vi "Inspect Modules.vi"(7 "Console Log in":refnum<class "Console Log.lvclass">, 8 "error in":errorcluster, 11 "Potting Procedure in":refnum<class "Potting Procedure.lvclass">) -> (0 "error out":errorcluster, 3 "Potting Procedure out":refnum<class "Potting Procedure.lvclass">, 5 "Console Log out":refnum<class "Console Log.lvclass">)   [LabVIEW 2011, in "Potting Procedure.lvclass"]
uses:
  Potting Procedure.lvclass
  Application Utilities/Console Log/Console Log.lvclass
  Type Definitions/Inspect Modules.ctl
  Type Definitions/Inspect Modules - Module.ctl
  Shared Components/Utils/Type Definitions/Multi-Fiducial Image.ctl
  Shared Components/Utils/Type Definitions/Physical Image.ctl
  Shared Components/Vec3d Class/Vec3d Class.lvclass
  <vilib>/vision/Image Controls.llb/IMAQ Image.ctl
  Shared Components/Utils/Type Definitions/Fiducial with Source.ctl
  Shared Components/Utils/Type Definitions/Fiducial Image.ctl
  Shared Components/Gantry Class/Gantry Class.lvclass
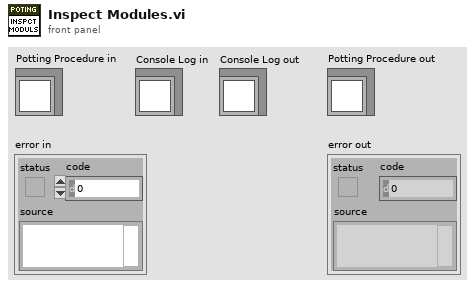
[diagram p1: front panel]
types:
  T1 = typedef "Inspect Modules.ctl" = cluster{"Has Been Run?":bool, "Module Positions":T2[]}
  T2 = typedef "Inspect Modules - Module.ctl" = cluster{"TBM-TBM":T3, "TBM-HDI":T3, "Address Pads":T3, "HDI Bond Pad References":T7[], "BBM Bond Pad References":T7[], "HV-HDI":T7, "HV-BBM":T7, "Chuck":i32, "Slot":i32, "Potting Selection":cluster{"HDI Bond Pads":bool[], "BBM Bond Pads":bool[], "TBM Inner":cluster{"Top":bool, "Left":bool, "Bottom":bool, "Right":bool}, "TBM Outer":cluster{"Top":bool, "Left":bool, "Bottom":bool, "Right":bool}, "Address Pads":cluster{"Top":bool, "Bottom":bool}, "High Voltage":cluster{"HDI":bool, "BBM":bool}}}
  T3 = typedef "Multi-Fiducial Image.ctl" = cluster{"Fiducial Image":T4, "Fiducials":cluster{"Selected Fiducial":T6, "fiducial name":string}[]}
  T4 = typedef "Physical Image.ctl" = cluster{"Image Position":refnum<class "Vec3d Class.lvclass">, "Image Reference":T5, "Field of View":cluster{"x(mm)":dbl, "y(mm)":dbl}}
  T5 = typedef "IMAQ Image.ctl" = refnum<image>
  T6 = typedef "Fiducial with Source.ctl" = cluster{"Fiducial Image Coordinate":refnum<class "Vec3d Class.lvclass">, "Fiducial Source":enum16{"Pattern Recognition", "User", "Error", "Default"}}
  T7 = typedef "Fiducial Image.ctl" = cluster{"Fiducial Image":T4, "Selected Fiducial":T6, "fiducial name":string}
  T8 = typedef "Inspect Fiducials.ctl" = cluster{"Has Been Run?":bool, "Module-Chuck Fiducials":cluster{"Fiducials-HDI":T7[], "Fiducials-BBM":T7[], "Chuck":i32, "Slot":i32}[]}
  T9 = cluster{"Fiducials-HDI":T7[], "Fiducials-BBM":T7[], "Chuck":i32, "Slot":i32}[]
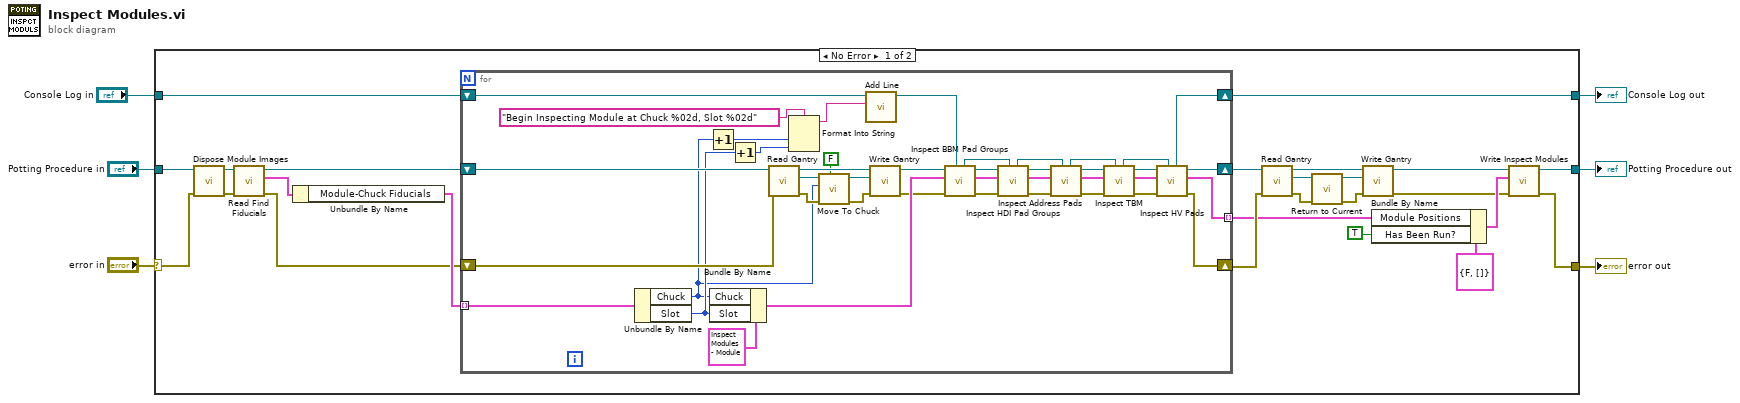
[diagram p0: block diagram]
diagram:
  n1 = case shown="No Error" "error in" {
    selector: "error in" -> [w8 w75]
    tunnel: [w14 w75] -> w5
    tunnel: [w28 w74] -> w3
    tunnel: "Potting Procedure in" -> [w11 w74]
    tunnel: "Console Log in" -> [w24 w73]
    tunnel: [w23 w73] -> w1
    frame No Error {
      n2 = call-dynamic "Dispose Module Images.vi"("error in"=w8, "Potting Procedure in"=w11) -> ("error out"=w9:errorcluster, "Potting Procedure out"=w10:refnum<class "Potting Procedure.lvclass">)  [unwired: 8 in]
      n3 = call-dynamic "Read Find Fiducials.vi"("error in (no error)"=w9, "Potting Procedure in"=w10) -> ("error out"=w7:errorcluster, "Find Fiducials"=w30:T8, "Potting Procedure out"=w31:refnum<class "Potting Procedure.lvclass">)  [unwired: 7 in]
      n4 = Unbundle By Name(w30) -> ("Module-Chuck Fiducials"=w29:T9)
      n5 = for {
        shift-right: [w34] -> w18
        shift-left: w31 -> [w62]
        shift-right: [w35] -> w16
        shift-left: w7 -> [w61]
        tunnel: w29 -> [w72] mode=indexing
        shift-right: [w36] -> w23
        shift-left: w24 -> [w53]
        tunnel: [w32] -> w13 mode=indexing
        n6 = Unbundle By Name(w72) -> ("Chuck"=w45:i32, "Slot"=w49:i32)
        n7 = Increment(x=w45) -> (x+1=w47:i32)
        n8 = Bundle By Name(cluster=T2 {"TBM-TBM"={"Fiducial Image"={"Image Position"=refnum, "Image Reference"=refnum, "Field of View"={"x(mm)"=0.0, "y(mm)"=0.0}}, "Fiducials"=[]}, "TBM-HDI"={"Fiducial Image"={"Image Position"=refnum, "Image Reference"=refnum, "Field of View"={"x(mm)"=0.0, "y(mm)"=0.0}}, "Fiducials"=[]}, "Address Pads"={"Fiducial Image"={"Image Position"=refnum, "Image Reference"=refnum, "Field of View"={"x(mm)"=0.0, "y(mm)"=0.0}}, "Fiducials"=[]}, "HDI Bond Pad References"=[], "BBM Bond Pad References"=[], "HV-HDI"={"Fiducial Image"={"Image Position"=refnum, "Image Reference"=refnum, "Field of View"={"x(mm)"=0.0, "y(mm)"=0.0}}, "Selected Fiducial"={"Fiducial Image Coordinate"=refnum, "Fiducial Source"=enum."Pattern Recognition"}, "fiducial name"=""}, "HV-BBM"={"Fiducial Image"={"Image Position"=refnum, "Image Reference"=refnum, "Field of View"={"x(mm)"=0.0, "y(mm)"=0.0}}, "Selected Fiducial"={"Fiducial Image Coordinate"=refnum, "Fiducial Source"=enum."Pattern Recognition"}, "fiducial name"=""}, "Chuck"=0, "Slot"=0, "Potting Selection"={"HDI Bond Pads"=[TRUE, TRUE, TRUE, TRUE, TRUE, TRUE, TRUE, TRUE, TRUE, TRUE, TRUE, TRUE, TRUE, TRUE, TRUE, TRUE], "BBM Bond Pads"=[TRUE, TRUE, TRUE, TRUE, TRUE, TRUE, TRUE, TRUE, TRUE, TRUE, TRUE, TRUE, TRUE, TRUE, TRUE, TRUE], "TBM Inner"={"Top"=TRUE, "Left"=TRUE, "Bottom"=TRUE, "Right"=TRUE}, "TBM Outer"={"Top"=TRUE, "Left"=TRUE, "Bottom"=TRUE, "Right"=TRUE}, "Address Pads"={"Top"=TRUE, "Bottom"=TRUE}, "High Voltage"={"HDI"=TRUE, "BBM"=TRUE}}} ("Module"), "Chuck"=w45, "Slot"=w49) -> (w65:T2)
        n9 = Increment(x=w49) -> (x+1=w48:i32)
        n10 = call-dynamic "Read Gantry.vi"("error in (no error)"=w61, "Potting Procedure in"=w62) -> ("error out"=w64:errorcluster, "Gantry"=w63:refnum<class "Gantry Class.lvclass">, "Potting Procedure out"=w58:refnum<class "Potting Procedure.lvclass">)  [unwired: 7 in]
        n11 = Format Into String(format string="Begin Inspecting Module at Chuck %02d, Slot %02d" ("initial string"), w47, w48) -> (resulting string=w51:string)  [unwired: 2 in, 1 out]
        n12 = call-dynamic "Move To Chuck.vi"("Move if Same"=FALSE, "error in"=w64, "Chuck"=w45, "Gantry in"=w63) -> ("error out"=w60:errorcluster, "Gantry out"=w59:refnum<class "Gantry Class.lvclass">)  [unwired: 6 in]
        n13 = call "Add Line.vi"("String"=w51, "Console Log in"=w53) -> ("Console Log out"=w52:refnum<class "Console Log.lvclass">)  [unwired: 8 in, 1 out]
        n14 = call-dynamic "Write Gantry.vi"("error in (no error)"=w60, "Gantry"=w59, "Potting Procedure in"=w58) -> ("error out"=w56:errorcluster, "Potting Procedure out"=w57:refnum<class "Potting Procedure.lvclass">)  [unwired: 7 in]
        n15 = call-dynamic "Inspect BBM Pad Groups.vi"("Console Log in"=w52, "error in"=w56, "Module Data In"=w65, "Potting Procedure in"=w57) -> ("error out"=w70:errorcluster, "Module Data Out"=w67:T2, "Potting Procedure out"=w71:refnum<class "Potting Procedure.lvclass">, "Console Log out"=w55:refnum<class "Console Log.lvclass">)  [unwired: 4 in]
        n16 = call "Inspect HDI Pad Groups.vi"("Console Log in"=w55, "error in"=w70, "Module Data In"=w67, "Potting Procedure in"=w71) -> ("error out"=w68:errorcluster, "Module Data Out"=w66:T2, "Potting Procedure out"=w69:refnum<class "Potting Procedure.lvclass">, "Console Log out"=w54:refnum<class "Console Log.lvclass">)  [unwired: 4 in]
        n17 = call "Inspect Address Pads.vi"("Console Log in"=w54, "error in"=w68, "Module Data In"=w66, "Potting Procedure in"=w69) -> ("error out"=w44:errorcluster, "Module Data Out"=w43:T2, "Potting Procedure out"=w42:refnum<class "Potting Procedure.lvclass">, "Console Log out"=w41:refnum<class "Console Log.lvclass">)  [unwired: 4 in]
        n18 = call "Inspect TBM.vi"("Console Log in"=w41, "error in"=w44, "Module Data In"=w43, "Potting Procedure in"=w42) -> ("error out"=w40:errorcluster, "Module Data Out"=w39:T2, "Potting Procedure out"=w38:refnum<class "Potting Procedure.lvclass">, "Console Log out"=w37:refnum<class "Console Log.lvclass">)  [unwired: 4 in]
        n19 = call "Inspect HV Pads.vi"("Console Log in"=w37, "error in"=w40, "Module Data In"=w39, "Potting Procedure in"=w38) -> ("error out"=w35:errorcluster, "Module Data Out"=w32:T2, "Potting Procedure out"=w34:refnum<class "Potting Procedure.lvclass">, "Console Log out"=w36:refnum<class "Console Log.lvclass">)  [unwired: 4 in]
      }
      n20 = call-dynamic "Read Gantry.vi"("error in (no error)"=w16, "Potting Procedure in"=w18) -> ("error out"=w19:errorcluster, "Gantry"=w20:refnum<class "Gantry Class.lvclass">, "Potting Procedure out"=w12:refnum<class "Potting Procedure.lvclass">)  [unwired: 7 in]
      n21 = call-dynamic "Return to Current.vi"("error in"=w19, "Gantry in"=w20) -> ("error out"=w21:errorcluster, "Gantry out"=w22:refnum<class "Gantry Class.lvclass">)  [unwired: 8 in]
      n22 = call-dynamic "Write Gantry.vi"("error in (no error)"=w21, "Gantry"=w22, "Potting Procedure in"=w12) -> ("error out"=w15:errorcluster, "Potting Procedure out"=w17:refnum<class "Potting Procedure.lvclass">)  [unwired: 7 in]
      n23 = Bundle By Name(cluster=T1 {"Has Been Run?"=FALSE, "Module Positions"=[]} ("Inspect Modules"), "Module Positions"=w13, "Has Been Run?"=TRUE) -> (w26:T1)
      n24 = call-dynamic "Write Inspect Modules.vi"("error in (no error)"=w15, "Inspect Modules"=w26, "Potting Procedure in"=w17) -> ("error out"=w14:errorcluster, "Potting Procedure out"=w28:refnum<class "Potting Procedure.lvclass">)  [unwired: 7 in]
    }
    frame Error {
    }
  }
  "error out" <- w5
  "Potting Procedure out" <- w3
  "Console Log out" <- w1
